vi "Switch to WiFi.vi"(8 "Error In":errorcluster, 10 "TCP Configuration":T5, 11 "LINX Resource":T1) -> (0 "Error Out":errorcluster, 3 "LINX Resource out":T1)   [LabVIEW 2019, in "LINXx.lvlib"]
doc: "Switch from serial connection to the LINX device to TCP communication. If TCP settings fail, VI continues with original serial connection.\nUse IP address 0.0.0.0 to use DHCP (router assigns address to board)"
uses:
  LINXx.lvlib
  <vilib>/MakerHub/LINX/Private/Device/Type Defs/TCP Config.ctl
  <vilib>/MakerHub/LINX/Private/Type Defs/LINX Ref.ctl
  <vilib>/MakerHub/LINX/Private/Type Defs/Platform.ctl
  <vilib>/MakerHub/LINX/Private/Type Defs/Interface.ctl
  <vilib>/MakerHub/LINX/Private/Device/Type Defs/LINX Device Config.ctl
  <vilib>/MakerHub/LINX/Private/Device/Type Defs/Channels.ctl
  <vilib>/Utility/error.llb/DialogType.ctl
  <vilib>/MakerHub/LINX/Public/Utilities/Open TCP.vi
  <vilib>/MakerHub/LINX/LMH-LINX.lvlib
  <vilib>/MakerHub/LINX/Private/Device/Device.lvlib
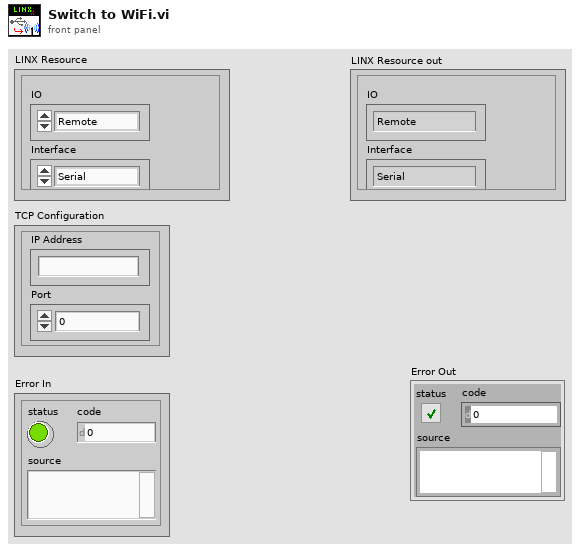
[diagram p1: front panel]
types:
  T1 = typedef "LMH-LINX.lvlib/LINX Ref.ctl" = cluster{"IO":T2, "Interface":T3, "LINX Device Config":T4}
  T2 = typedef "LMH-LINX.lvlib/Platform.ctl" = enum16{"Remote", "Local"}
  T3 = typedef "LMH-LINX.lvlib/Interface.ctl" = enum16{"Serial", "TCP"}
  T4 = typedef "LMH-LINX.lvlib/Device.lvlib/LINX Device Config.ctl" = cluster{"Interface":T3, "COM Port":refnum<visa-resource-name>, "TCP Configuration":T5, "Device Family":u8, "Device ID":u8, "Device Name":string, "TCP Ref":refnum<k5>, "Channels":T6}
  T5 = typedef "LMH-LINX.lvlib/Device.lvlib/TCP Config.ctl" = cluster{"IP Address":string, "Port":u16}
  T6 = typedef "LMH-LINX.lvlib/Channels.ctl" = cluster{"DI":u8[], "DO":u8[], "AI":u8[], "AO":u8[], "PWM":u8[], "QE":u8[], "UART":u8[], "I2C 2":u8[], "SPI":u8[], "CAN":u8[], "Servo":u8[], "AI Ref (V)":dbl, "AI Resolution (Bits)":u8, "AO Ref (V)":dbl, "AO Resolution (Bits)":u8}
  T7 = typedef "DialogType.ctl" = u16
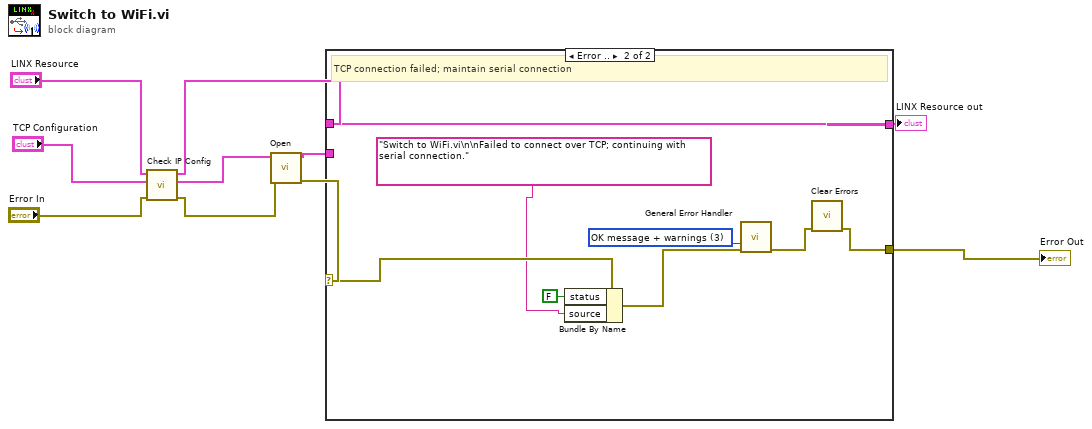
[diagram p0: block diagram]
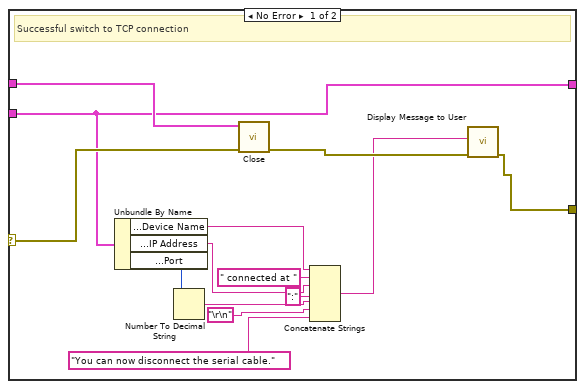
[diagram p2: hidden frame]
diagram:
  n1 = call "Check IP Config.vi"("Error In"="Error In", "TCP Configuration"="TCP Configuration", "LINX Resource"="LINX Resource") -> ("error out"=w5:errorcluster, "TCP Config out"=w1:T5, "LINX Resource Out"=w3:T1)  [unwired: 6 in]
  n2 = call-poly <vilib>:"Open.vi"("Error In"=w5, "TCP Configuration"=w1) -> ("Error Out"=w10:errorcluster, "LINX Resource"=w9:T1)  [unwired: 7 in, 1 out]
  n3 = case shown="Error .." w10 {
    selector: w10 -> [w23 w31]
    tunnel: w3 -> [w24 w32]
    tunnel: [w22 w32] -> w8
    tunnel: w9 -> [w22 _]
    tunnel: [w12 w25] -> w7
    frame No Error {
      # "Successful switch to TCP connection"
      n4 = Unbundle By Name(w22) -> ("LINX Device Config.Device Name"=w21:string, "LINX Device Config.TCP Configuration.IP Address"=w19:string, "LINX Device Config.TCP Configuration.Port"=w17:u16)
      n5 = Number To Decimal String(number=w17) -> (decimal integer string=w16:string)  [unwired: 1 in]
      n6 = call <vilib>:"Close.vi"("Error In"=w23, "LINX Resource"=w24) -> ("Error Out"=w13:errorcluster)  [unwired: 9 in]
      n7 = Concatenate Strings(w21, " connected at " ("string"), w19, ":" ("string"), w16, "\r\n", "You can now disconnect the serial cable." ("string")) -> (w11:string)
      n8 = call "Display Message to User"("error in (no error)"=w13, "Message"=w11) -> ("error out"=w12:errorcluster)  [unwired: 8 in, 1 out]
    }
    frame Error {
      w28 = T7 3 items=["no dialog", "OK message", "continue or stop message", "OK message + warnings", "continue/stop + warnings"] ("type of dialog (OK msg:1)")
      # "TCP connection failed; maintain serial connection"
      n9 = Bundle By Name(cluster=w31, "status"=FALSE, "source"="Switch to WiFi.vi\n\nFailed to connect over TCP; continuing with serial connection." ("string")) -> (w27:errorcluster)
      n10 = call <vilib>:"General Error Handler.vi"("type of dialog (OK msg:1)"=w28, "error in (no error)"=w27) -> ("error out"=w26:errorcluster)  [unwired: 9 in, 4 out]
      n11 = call <vilib>:"Clear Errors.vi"("error in (no error)"=w26) -> ("error out"=w25:errorcluster)  [unwired: 5 in, 1 out]
    }
  }
  "Error Out" <- w7
  "LINX Resource out" <- w8
